vi "Harmonic Analyzer Measurement.vi"() -> ()   [LabVIEW 2020]
doc: "Given an input signal, finds the fundamental frequency and its harmonics, and computes Total Harmonic Distortion (THD). \n\nYou can further control the measurement by restricting the number of harmonics used to compute THD and by including or excluding frequencies that may have aliased (ideal-like square waves have high frequency harmonics that appear to have aliased to lower frequencies). If you are interested in a particular test frequency, you can specify it using the advanced search criteria of approximate fundamental frequency and percent search."
uses:
  <vilib>/measure/matone.llb/Harmonic Distortion Analyzer.vi
  <vilib>/measure/NI_MAPro.lvlib
panel:
  out "measurement info comments":string
  in  "advanced search":T1={"approx freq. (optional)"=-1.0, "search (+/- % of Fsampl.)"=5.0} {"search (+/- % of Fsampl.)" format="%#.6g"; "approx freq. (optional)" format="%#.6g"}
  in  "highest harmonic":i32=25
  in  "Exclude aliased harmonics":bool
  out "frequency (Hz)":dbl=1234.89 format="%#.6g"
  in  "export mode":T2(ring)=enum."input signal"
  in  "noise (bitVolt)":dbl(slide)=-16.018367346938778
  in  "Block size":i32=1024
  out "THD (%)":dbl=0.01982415763775073 format="%0.6f"
  out "exported signal spectrum (dBV)":T3(graph)
  in  "1mV at 60 Hz":bool
  in  "Stop":bool
  out "exported time signal":waveform(dbl)(graph)
  in  "amplitude (V)":dbl=1.0 format="%#.6g"
  in  "signal frequency (Hz)":dbl=1234.89 format="%#.6g"
  in  "Fs (Hz)":dbl=51200.0 format="%0.0f"
  # "Overview: Demonstrates the use of the Harmonic Distortion Analyzer VI to find the fundamental tone and associated THD (Total Harmonic Distortion).\nRequirements: LabVIEW Full Development System\nInstructions:\n1. Run the VI and change the noise slider and note how noise affects the THD (%) measurement.\n2. Use the export mode to select the signal to export. Try the \"harmonic only\" value to view only the harmonics of the distorted test signal.\n3. Click Stop to stop the VI."
  # "Input Signal"
  # "Analysis Results"
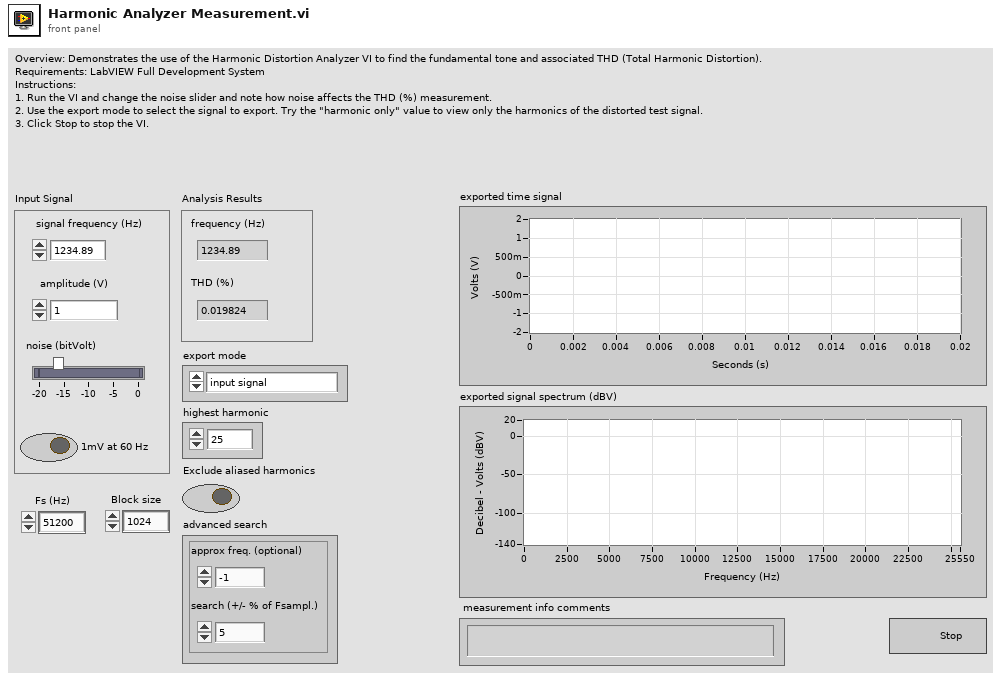
[diagram p1: front panel]
types:
  T1 = cluster{"approx freq. (optional)":dbl, "search (+/- % of Fsampl.)":dbl}
  T2 = enum16{"none", "input signal", "fundamental signal", "residual signal", "harmonics only", "noise and spurs"}
  T3 = cluster{"f0":dbl, "df":dbl, "dB Spectrum (Hann)":dbl[]}
  T4 = cluster{"uncertainty":dbl, "Warning":bool, "comments":string}
  T5 = cluster{"exported time signal":waveform(dbl), "exported spectrum (dB)":cluster{"f0":dbl, "df":dbl, "dB Spectrum (Hann)":dbl[]}}
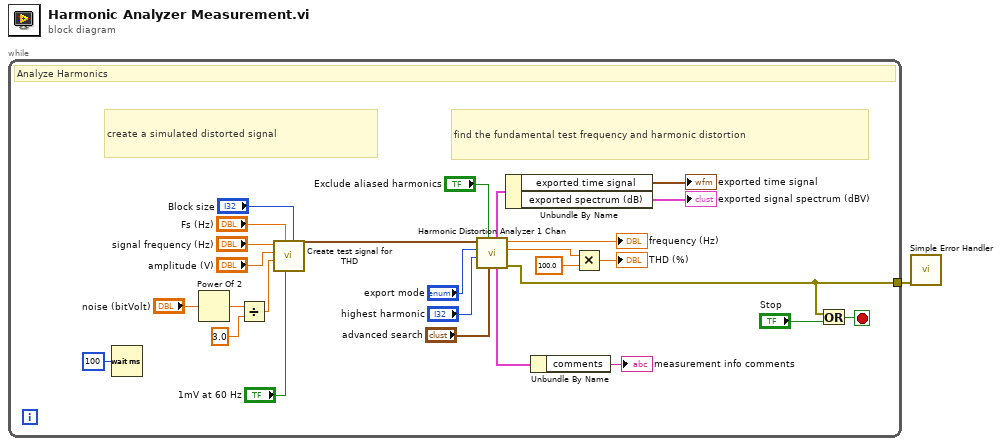
[diagram p0: block diagram]
diagram:
  n1 = while {
    tunnel: [w5] -> w1
    stop <- w6 stop-if-true
    # "find the fundamental test frequency and harmonic distortion"
    # "create a simulated distorted signal"
    # "Analyze Harmonics"
    n2 = Wait (ms)(milliseconds to wait=u32 100 ("f")) -> ()  [unwired: 1 out]
    n3 = Power Of 2(x="noise (bitVolt)") -> (2^x=w26:dbl)
    n4 = Divide(x=w26, y=3.0) -> (x/y=w24:dbl)
    n5 = call "Create test signal for THD.vi"("block size"="Block size", "1mV at 60 Hz"="1mV at 60 Hz", "sampling frequency (Hz)"="Fs (Hz)", "noise level (Vrms)"=w24, "fundamental amplitude"="amplitude (V)", "fundamental frequency (Hz)"="signal frequency (Hz)") -> ("Test signal"=w11:waveform(dbl))  [unwired: 5 in]
    n6 = call-poly <vilib>:"Harmonic Distortion Analyzer 1 Chan.vi"("advanced search"="advanced search", "stop search at Nyquist"="Exclude aliased harmonics", "highest harmonic"="highest harmonic", "export mode"="export mode", "signal in"=w11) -> ("error out"=w5:errorcluster, "THD"=w19:dbl, "detected fundamental frequency"=→"frequency (Hz)":dbl, "measurement info"=w8:T4, "exported signals"=w14:T5)  [unwired: 1 in, 1 out]
    n7 = Unbundle By Name(w14) -> ("exported time signal"=→"exported time signal":waveform(dbl), "exported spectrum (dB)"=→"exported signal spectrum (dBV)":T3)
    n8 = Unbundle By Name(w8) -> ("comments"=→"measurement info comments":string)
    n9 = Multiply(x=w19, y=100.0) -> (x*y=→"THD (%)":dbl)
    n10 = Or(x=w5, y="Stop") -> (x .or. y?=w6:bool)
  }
  n11 = call <vilib>:"Simple Error Handler.vi"("error in (no error)"=w1) -> ()  [unwired: 4 in, 5 out]
